vi "Panel.vi"(11 "DblControlEditorPanel in":refnum<class "DblControlEditorPanel.lvclass">) -> ()   [LabVIEW 2020, in "VolatusGUIControls.lvlib" / "DblControlEditorPanel.lvclass"]
uses:
  DblControlEditorPanel.lvclass
  C:/dev/lv20CE/relink/volatus-gui-controls/VolatusGUIEditorCore/ElementEditorPanel/ElementEditorPanel.lvclass
  C:/dev/lv20CE/relink/lv-oopanel/OOPanel/Panel/Panel.lvclass
  lv-oopanel/OOPanel/Panel/Basic UI State.ctl
  lv-autocomplete/AutoComplete/AutoComplete/AutoComplete.lvclass/AutoComplete.ctl
  DblControlEditorPanel.lvclass/DblControlEditorPanel.ctl
  lv-autocomplete/AutoComplete/Launch Autocomplete Handler.vi
  lv-autocomplete/AutoComplete/AutoComplete/AutoComplete.lvclass
  lv-oopanel/OOPanel/Panel/Panel.lvclass
  lv-oopanel/OOPanel/OOPanel.lvlib
  VolatusGUIEditorCore/ElementEditorPanel/ElementEditorPanel.lvclass
  VolatusGUIEditorCore/VolatusGUIEditorCore.lvlib
panel:
  in  "Height":u16
  in  "Decimals":u8
  in  "BG Color":u32(colorbox)
  in  "Font Color":u32(colorbox)
  in  "Top":i32
  in  "Left":i32
  in  "Width":u16
  in  "Label Text Color":u32(colorbox) caption="Color"
  in  "Label Visible":bool caption="Visible"
  in  "Label":string
  in  "Channel":string
  # "Label"
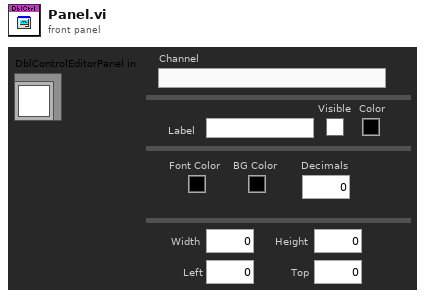
[diagram p1: front panel]
types:
  T1 = typedef "OOPanel.lvlib/Panel.lvclass/Basic UI State.ctl" = enum16{"Init", "Run", "Close"}
  T2 = typedef "VolatusGUIEditorCore.lvlib/ElementEditorPanel.lvclass/Incoming Events.ctl" = cluster{"Update Control":refnum<user-event>}
  T3 = typedef "OOPanel.lvlib/Panel.lvclass/Panel Events.ctl" = cluster{"Visbility":refnum<user-event>, "Close":refnum<user-event>}
  T4 = typedef "VolatusGUIControls.lvlib/DblControlEditorPanel.lvclass/Props.ctl" = cluster{"JSON":T5, "Label":T6, "Position":T7, "Width":u16, "Height":u16, "Numeric Text":T8}
  T5 = typedef "VolatusGUIControls.lvlib/DblControlEditorPanel.lvclass/JSON Props.ctl" = cluster{"Channel":string}
  T6 = typedef "VolatusGUIEditorCore.lvlib/Label Props.ctl" = cluster{"Text":string, "Text Color":u32, "Visible":bool}
  T7 = typedef "VolatusGUIEditorCore.lvlib/Position Props.ctl" = cluster{"Left":i32, "Top":i32}
  T8 = typedef "VolatusGUIEditorCore.lvlib/Numeric Text Props.ctl" = cluster{"Font Color":u32, "BG Color":u32, "Format String":string}
  T9 = typedef "OOPanel.lvlib/Visibility State.ctl" = enum16{"Idle", "Closed", "Hidden", "Visible", "Subpanel", "Hidden Subpanel"}
  T10 = cluster{"Label":string, "Label Text Color":u32, "Label Visible":bool}
  T11 = cluster{"Font Color":u32, "BG Color":u32, "Format String":string}
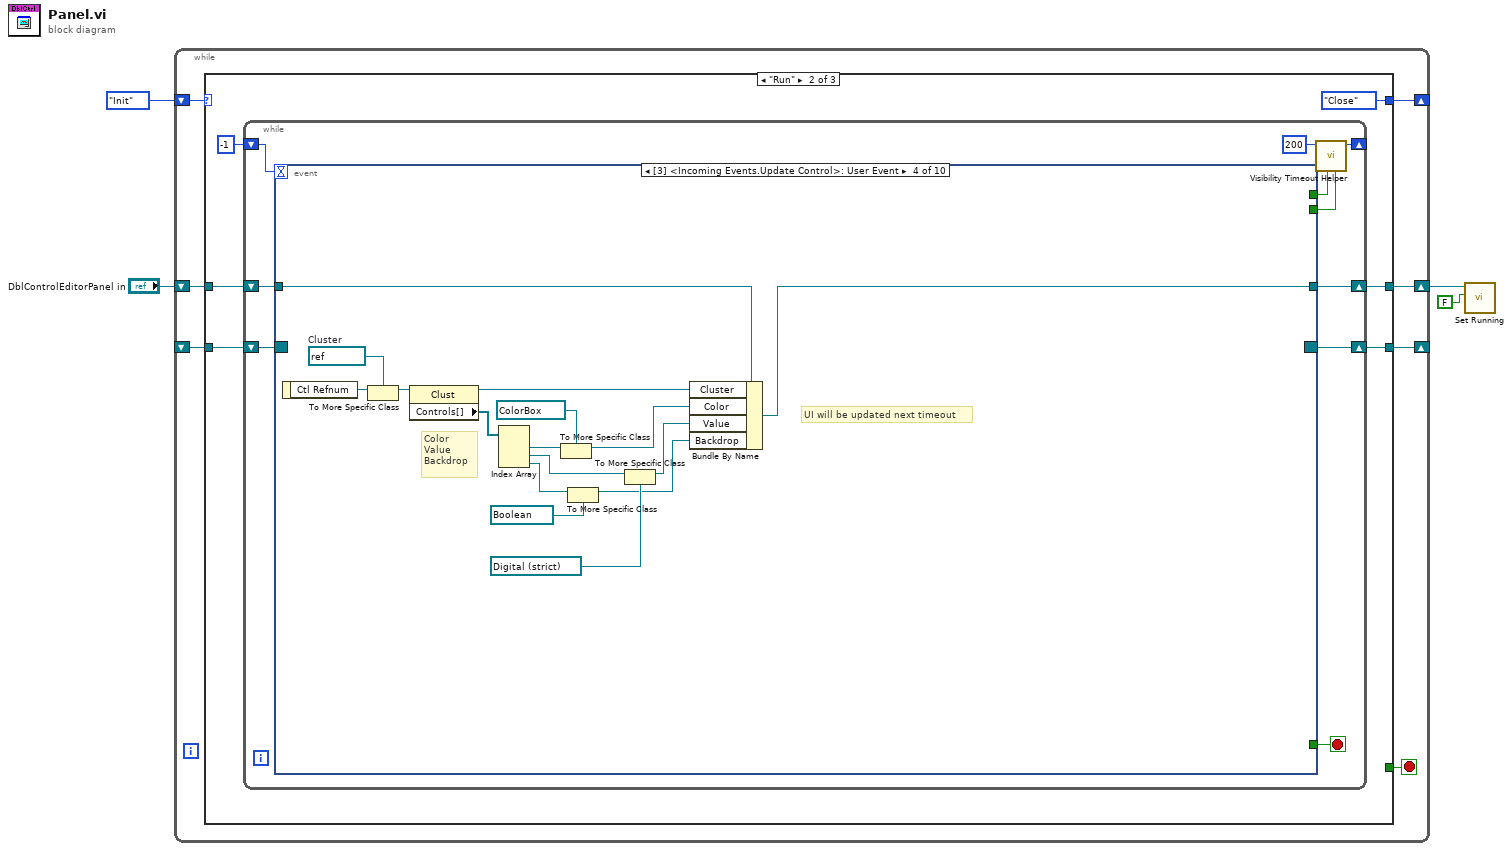
[diagram p0: block diagram]
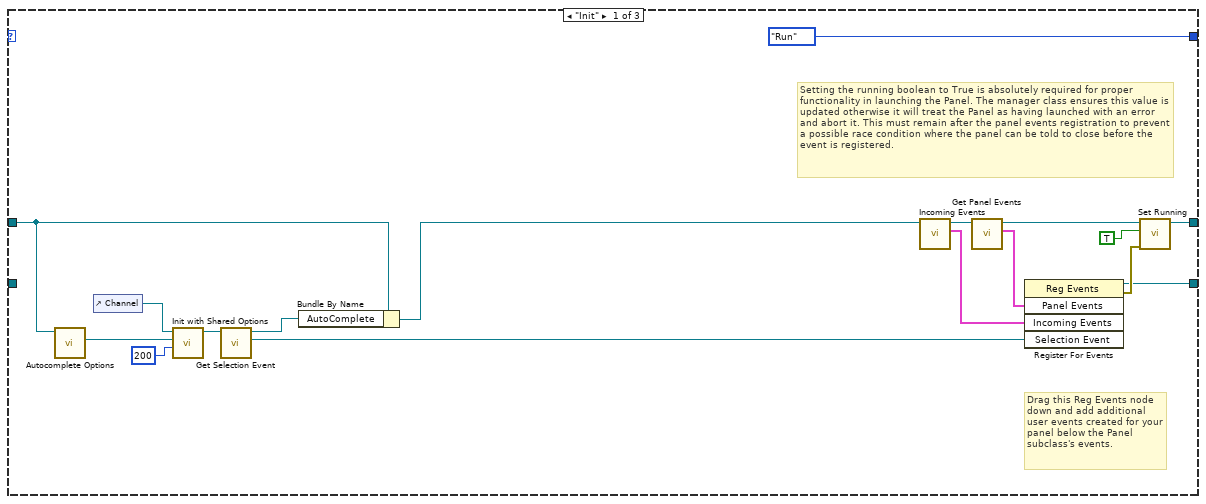
[diagram p2: hidden frame]
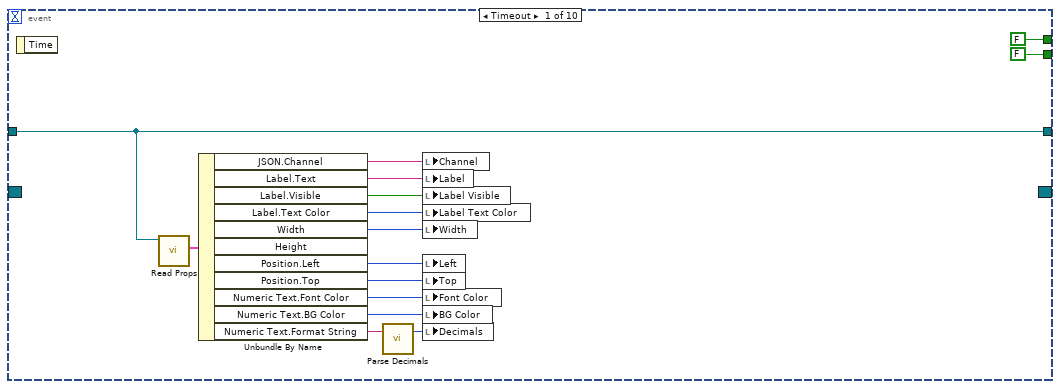
[diagram p3: hidden frame]
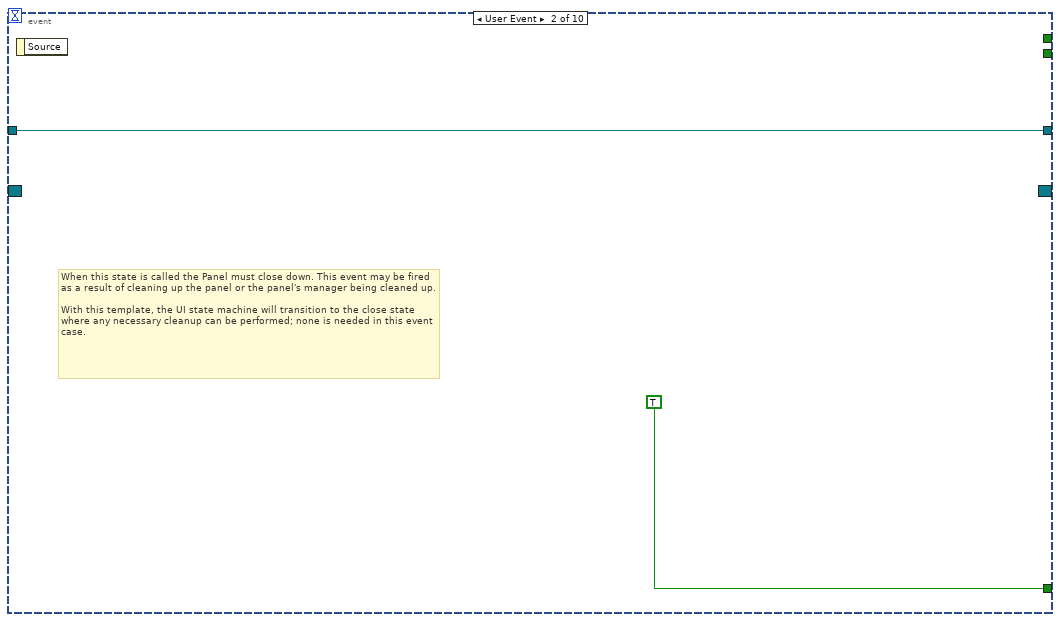
[diagram p4: hidden frame]
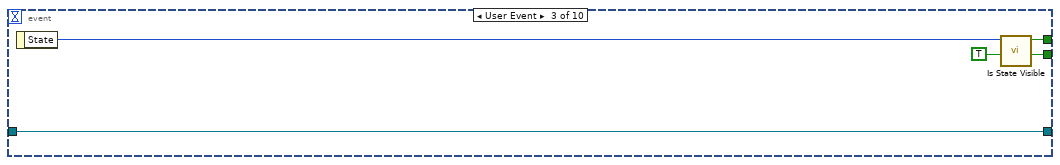
[diagram p5: hidden frame]
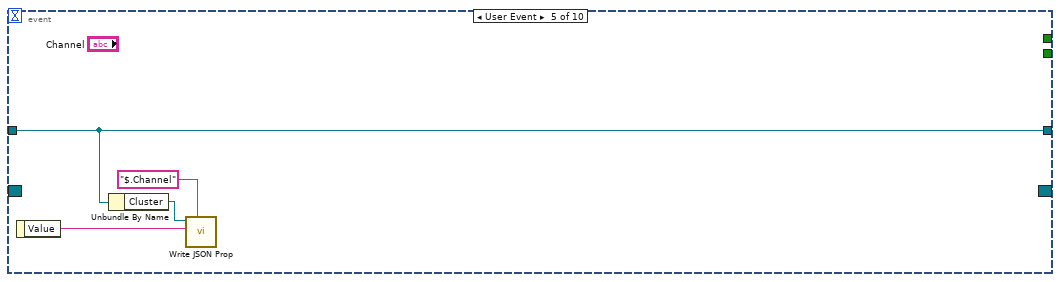
[diagram p6: hidden frame]
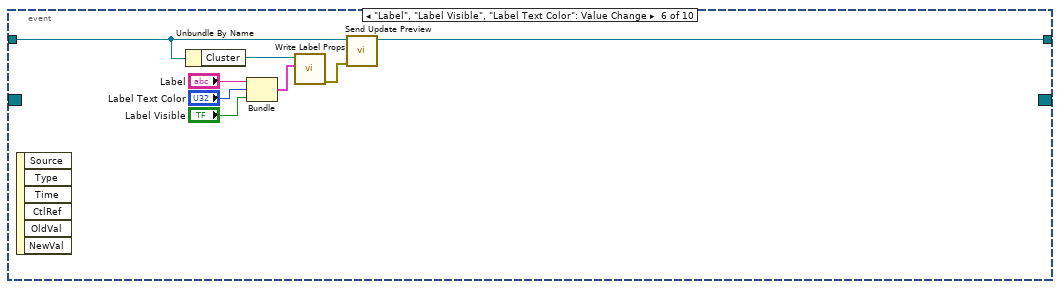
[diagram p7: hidden frame]
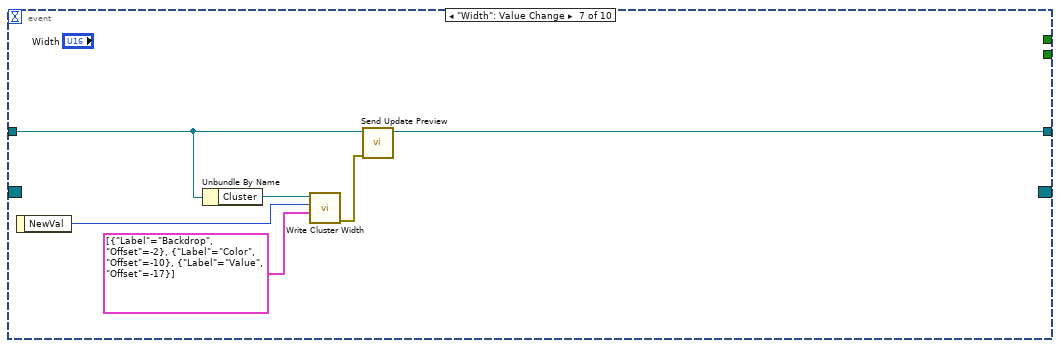
[diagram p8: hidden frame]
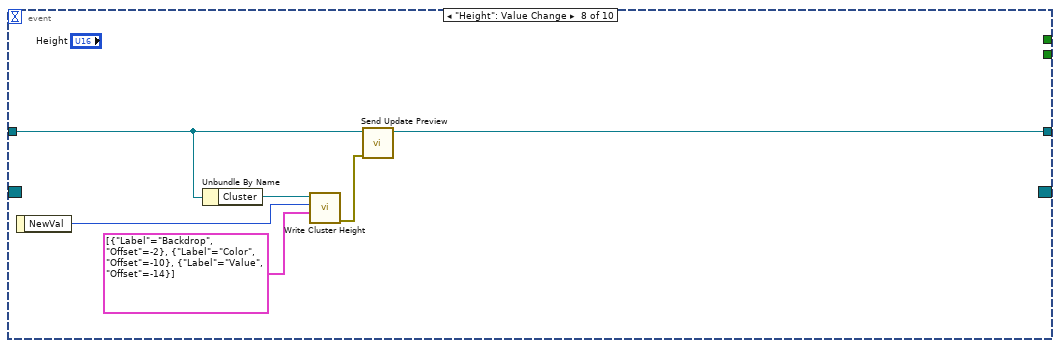
[diagram p9: hidden frame]
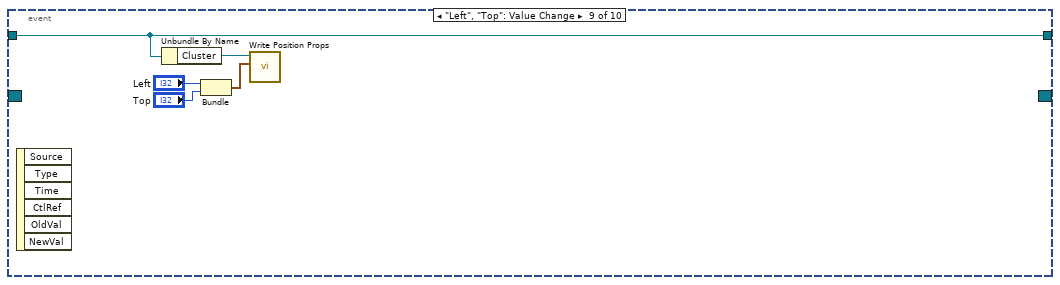
[diagram p10: hidden frame]
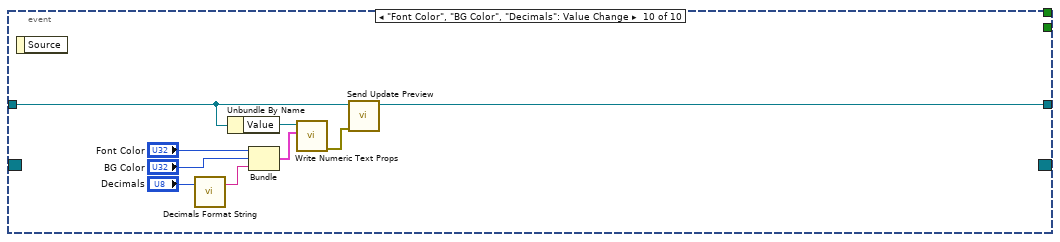
[diagram p11: hidden frame]
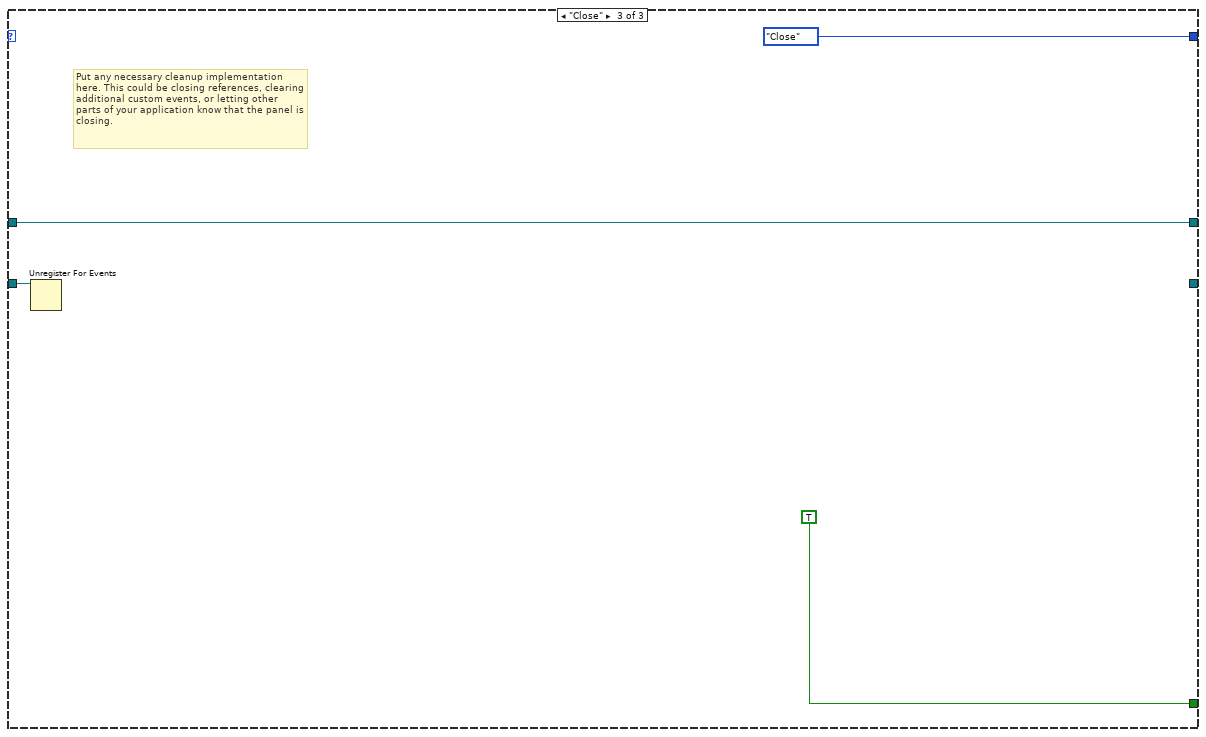
[diagram p12: hidden frame]
diagram:
  n1 = while {
    shift-right: [w10] -> _
    shift-left: _ -> [w11]
    shift-right: [w8] -> _
    shift-left: Basic_UI_State."Init" ("Basic UI State") -> [w9]
    shift-right: [w6] -> w4
    shift-left: "DblControlEditorPanel in" -> [w5]
    stop <- w7 stop-if-true
    n2 = case shown="\"Run\"" w9 {
      tunnel: w11 -> [_ w34 w121]
      tunnel: [w25 w32 _] -> w10
      tunnel: [Basic_UI_State."Run" ("Basic UI State") Basic_UI_State."Close" ("Basic UI State") Basic_UI_State."Close" ("Basic UI State")] -> w8
      tunnel: [_ _ TRUE] -> w7
      tunnel: [w24 w29 w120] -> w6
      tunnel: w5 -> [w15 w30 w120]
      frame "Init" {
        # "Setting the running boolean to True is absolutely required for proper functionality in launching the Panel. The manager class ensures this value is updated otherwise it will treat the Panel as having launched with an error and abort it. This must remain after the panel events registration to prevent a possible race condition where the panel can be told to close before the event is registered."
        # "Drag this Reg Events node down and add additional user events created for your panel below the Panel subclass's events."
        n3 = call "Autocomplete Options.vi"("ElementEditorPanel in"=w15) -> ("Autocomplete Options"=w19:refnum<class "Shared Options.lvclass">)  [unwired: 10 in]
        n4 = control-ref of="Channel"() -> (w14:refnum<vi>)
        n5 = call "Init with Shared Options.vi"("Height (200)"=i16 200, "Shared Options"=w19, "Str Refnum"=w14) -> ("AutoComplete out"=w17:refnum<class "AutoComplete.lvclass">)  [unwired: 7 in, 1 out]
        n6 = call "Get Selection Event.vi"("AutoComplete in"=w17) -> ("Selection Event"=w16:refnum<user-event>, "AutoComplete"=w12:refnum<class "AutoComplete.lvclass">)  [unwired: 9 in]
        n7 = Bundle By Name(cluster=w15, "AutoComplete"=w12) -> (w13:refnum<class "DblControlEditorPanel.lvclass">)
        n8 = call "Incoming Events.vi"("ElementEditorPanel in"=w13) -> ("Incoming Events"=w21:T2, "ElementEditorPanel out"=w20:refnum<class "DblControlEditorPanel.lvclass">)  [unwired: 9 in]
        n9 = call "Get Panel Events.vi"("Panel in"=w20) -> ("Panel Events"=w22:T3, "Panel out"=w23:refnum<class "DblControlEditorPanel.lvclass">)  [unwired: 8 in, 1 out]
        n10 = register-events(w22, w21, w16) -> (reference out=w25:refnum<event-registration>, error out=w27:errorcluster)  [unwired: 2 in]
        n11 = call "Set Running.vi"("error in (no error)"=w27, "Running"=TRUE, "Panel in"=w23) -> ("Panel out"=w24:refnum<class "DblControlEditorPanel.lvclass">)  [unwired: 7 in, 1 out]
      }
      frame "Run" {
        n12 = while {
          shift-right: [w40] -> w32
          shift-left: w34 -> [w41]
          shift-right: [w43] -> _
          shift-left: -1 ("Timeout") -> [w42]
          shift-right: [w35] -> w29
          shift-left: w30 -> [w36]
          stop <- w37 stop-if-true
          n13 = event shown="[3] <Incoming Events.Update Control>: User Event" {
            selector: w41 -> [_ _ _ _ _ _ _ _ _ _]
            dyn-events: [_ _ _ _ _ _ _ _ _ _] -> w40
            timeout: w42 -> [_ _ _ _ _ _ _ _ _ _]
            tunnel: [FALSE _ w64 _ _ _ _ _ _ _] -> w39
            tunnel: [FALSE _ TRUE _ _ _ _ _ _ _] -> w38
            tunnel: [_ TRUE _ _ _ _ _ _ _ _] -> w37
            tunnel: w36 -> [w46 w60 w62 w81 w85 w92 w99 w105 w110 w119]
            tunnel: [w46 w60 w62 w69 w85 w93 w98 w104 w110 w118] -> w35
            event Timeout {
              n14 = event-data() -> ()  [unwired: 1 in, 1 out]
              n15 = call "Read Props.vi"("DblControlEditorPanel in"=w46) -> ("Props"=w57:T4)  [unwired: 9 in, 1 out]
              n16 = Unbundle By Name(w57) -> ("JSON.Channel"=w56:string, "Label.Text"=w55:string, "Label.Visible"=w54:bool, "Label.Text Color"=w53:u32, "Width"=w52:u16, "Position.Left"=w51:i32, "Position.Top"=w50:i32, "Numeric Text.Font Color"=w49:u32, "Numeric Text.BG Color"=w48:u32, "Numeric Text.Format String"=w47:string)  [unwired: 1 out]
              n17 = call "Parse Decimals.vi"("Format String"=w47) -> ("Decimals"=w45:u8)  [unwired: 6 in]
              n18 = local write "Channel"(w56) -> ()
              n19 = local write "Label"(w55) -> ()
              n20 = local write "Label Visible"(w54) -> ()
              n21 = local write "Label Text Color"(w53) -> ()
              n22 = local write "Width"(w52) -> ()
              n23 = local write "Left"(w51) -> ()
              n24 = local write "Top"(w50) -> ()
              n25 = local write "Font Color"(w49) -> ()
              n26 = local write "BG Color"(w48) -> ()
              n27 = local write "Decimals"(w45) -> ()
            }
            event User Event {
              # "When this state is called the Panel must close down. This event may be fired as a result of cleaning up the panel or the panel's manager being cleaned up.\n\nWith this template, the UI state machine will transition to the close state where any necessary cleanup can be performed; none is needed in this event case."
              n28 = event-data() -> ()  [unwired: 1 in, 1 out]
            }
            event User Event {
              n29 = event-data() -> ("State"=w65:T9)  [unwired: 1 in]
              n30 = call "Is State Visible.vi"("Visibility"=w65) -> ("Visible"=w64:bool)  [unwired: 10 in]
            }
            event User Event {
              w79 = refnum<vi> refnum  # Cluster
              # "UI will be updated next timeout"
              # "Color\nValue\nBackdrop"
              n31 = event-data() -> ("Ctl Refnum"=w80:refnum<vi>)  [unwired: 1 in]
              n32 = To More Specific Class(target class=w79, reference=w80) -> (specific class reference=w78:refnum<vi>)  [unwired: 1 in, 1 out]
              n33 = property class="Clust"(reference=w78) -> (reference out=w72:refnum<vi>, "Controls[]"=w77:refnum<vi>[])  [unwired: 1 in, 1 out]
              n34 = Index Array(array=w77) -> (element #1=w76:refnum<vi>, element #2=w75:refnum<vi>, element #3=w68:refnum<vi>)  [unwired: 3 in]
              n35 = To More Specific Class(target class=refnum<vi> refnum ("Color"), reference=w76) -> (specific class reference=w71:refnum<vi>)  [unwired: 1 in, 1 out]
              n36 = To More Specific Class(target class=refnum<vi> refnum ("Backdrop"), reference=w68) -> (specific class reference=w66:refnum<vi>)  [unwired: 1 in, 1 out]
              n37 = To More Specific Class(target class=refnum<vi> refnum ("Value"), reference=w75) -> (specific class reference=w70:refnum<vi>)  [unwired: 1 in, 1 out]
              n38 = Bundle By Name(cluster=w81, "Cluster"=w72, "Color"=w71, "Value"=w70, "Backdrop"=w66) -> (w69:refnum<class "DblControlEditorPanel.lvclass">)
            }
            event User Event {
              n39 = event-data() -> ("Value"=w82:string)  [unwired: 1 in]
              n40 = Unbundle By Name(w85) -> ("Cluster"=w84:refnum<vi>)
              n41 = call "Write JSON Prop.vi"("JSON Path"="$.Channel" ("$Path or Item Name"), "Value"=w82, "Ctl Refnum in"=w84) -> ()  [unwired: 7 in, 2 out]
            }
            event "Label", "Label Visible", "Label Text Color": Value Change {
              n42 = event-data() -> ()  [unwired: 1 in, 6 out]
              n43 = Unbundle By Name(w92) -> ("Cluster"=w88:refnum<vi>)
              n44 = Bundle("Label"="Label", "Label Text Color"="Label Text Color", "Label Visible"="Label Visible") -> (w87:T10)  [unwired: 1 in]
              n45 = call "Write Label Props.vi"("Label Props"=w87, "Ctl Refnum in"=w88) -> ("error out"=w86:errorcluster)  [unwired: 8 in, 1 out]
              n46 = call "Send Update Preview.vi"("error in (no error)"=w86, "ElementEditorPanel in"=w92) -> ("ElementEditorPanel out"=w93:refnum<class "DblControlEditorPanel.lvclass">)  [unwired: 8 in, 1 out]
            }
            event "Width": Value Change {
              n47 = event-data() -> ("NewVal"=w96:u16)  [unwired: 1 in]
              n48 = Unbundle By Name(w99) -> ("Cluster"=w95:refnum<vi>)
              n49 = call "Write Cluster Width.vi"("Nested Offsets (None)"=cluster{"Label":string, "Offset":i32}[] [{"Label"="Backdrop", "Offset"=-2}, {"Label"="Color", "Offset"=-10}, {"Label"="Value", "Offset"=-17}], "Width"=w96, "Cluster in"=w95) -> ("error out"=w94:errorcluster)  [unwired: 7 in, 1 out]
              n50 = call "Send Update Preview.vi"("error in (no error)"=w94, "ElementEditorPanel in"=w99) -> ("ElementEditorPanel out"=w98:refnum<class "DblControlEditorPanel.lvclass">)  [unwired: 8 in, 1 out]
            }
            event "Height": Value Change {
              n51 = event-data() -> ("NewVal"=w102:u16)  [unwired: 1 in]
              n52 = Unbundle By Name(w105) -> ("Cluster"=w101:refnum<vi>)
              n53 = call "Write Cluster Height.vi"("Nested Offsets (None)"=cluster{"Label":string, "Offset":i32}[] [{"Label"="Backdrop", "Offset"=-2}, {"Label"="Color", "Offset"=-10}, {"Label"="Value", "Offset"=-14}], "Height"=w102, "Cluster in"=w101) -> ("error out"=w100:errorcluster)  [unwired: 7 in, 1 out]
              n54 = call "Send Update Preview.vi"("error in (no error)"=w100, "ElementEditorPanel in"=w105) -> ("ElementEditorPanel out"=w104:refnum<class "DblControlEditorPanel.lvclass">)  [unwired: 8 in, 1 out]
            }
            event "Left", "Top": Value Change {
              n55 = event-data() -> ()  [unwired: 1 in, 6 out]
              n56 = Unbundle By Name(w110) -> ("Cluster"=w107:refnum<vi>)
              n57 = Bundle("Left"="Left", "Top"="Top") -> (w106:cluster{"Left":i32, "Top":i32})  [unwired: 1 in]
              n58 = call "Write Position Props.vi"("Position Props"=w106, "Ctl Refnum in"=w107) -> ()  [unwired: 8 in, 2 out]
            }
            event "Font Color", "BG Color", "Decimals": Value Change {
              n59 = event-data() -> ()  [unwired: 1 in, 1 out]
              n60 = call "Decimals Format String.vi"("Decimals"="Decimals") -> ("Format String"=w114:string)  [unwired: 6 in]
              n61 = Unbundle By Name(w119) -> ("Value"=w113:refnum<vi>)
              n62 = Bundle("Font Color"="Font Color", "BG Color"="BG Color", "Format String"=w114) -> (w112:T11)  [unwired: 1 in]
              n63 = call "Write Numeric Text Props.vi"("Numeric Text Props"=w112, "Control in"=w113) -> ("error out"=w111:errorcluster)  [unwired: 8 in, 1 out]
              n64 = call "Send Update Preview.vi"("error in (no error)"=w111, "ElementEditorPanel in"=w119) -> ("ElementEditorPanel out"=w118:refnum<class "DblControlEditorPanel.lvclass">)  [unwired: 8 in, 1 out]
            }
          }
          n65 = call "Visibility Timeout Helper.vi"("Update?"=w38, "Use Timeout?"=w39, "Visible Timeout mS"=200) -> ("Timeout"=w43:i32)  [unwired: 8 in]
        }
      }
      frame "Close" {
        # "Put any necessary cleanup implementation here. This could be closing references, clearing additional custom events, or letting other parts of your application know that the panel is closing."
        n66 = Unregister For Events(event registration refnum=w121) -> ()  [unwired: 1 in, 1 out]
      }
    }
  }
  n67 = call "Set Running.vi"("Running"=FALSE, "Panel in"=w4) -> ()  [unwired: 8 in, 2 out]
